vi "GetAllLibraries.vi"(8 "error in (no error)":errorcluster) -> (0 "error out":errorcluster, 3 "Lvlib paths":path[](array[path]))   [LabVIEW 2023, in "CICD.lvlib"]
uses:
  CICD.lvlib
  <userlib>/_OpenG.lib/file/file.llb/openg_file.lvlib
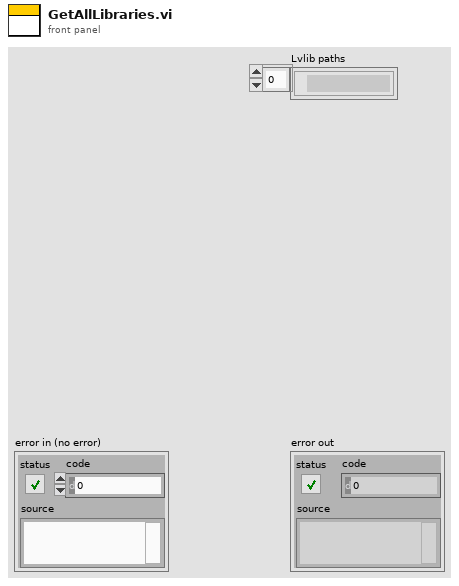
[diagram p1: front panel]
types:
  T1 = typedef "CICD.lvlib/CICDPathConfigs.ctl" = cluster{"GlobalIncludePaths":path[], "GlobalExcludePaths":path[], "BuildSpecsIncludePaths":path[], "ActualDepsIncludePaths":path[], "WorkspacePath":path, "SourceFolderPaths":path[]}
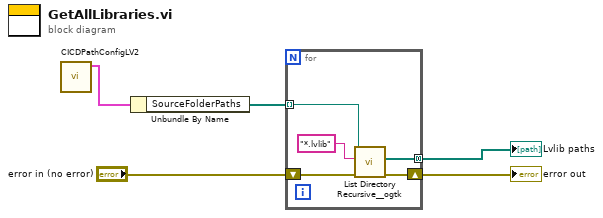
[diagram p0: block diagram]
diagram:
  n1 = call "CICDPathConfigLV2.vi"() -> ("CICD Path Config Out"=w1:T1)  [unwired: 11 in]
  n2 = Unbundle By Name(w1) -> ("SourceFolderPaths"=w4:path[])
  n3 = for {
    tunnel: [w10] -> w2 mode=concatenating
    shift-right: [w8] -> w3
    shift-left: "error in (no error)" -> [w9]
    tunnel: w4 -> [w6] mode=indexing
    n4 = call <userlib>:"List Directory Recursive__ogtk.vi"("error in (no error)"=w9, "pattern"="*.lvlib", "Path"=w6) -> ("error out"=w8:errorcluster, "file paths"=w10:path[])  [unwired: 5 in, 2 out]
  }
  "error out" <- w3
  "Lvlib paths" <- w2
